vi "Insert image into excel.vi"() -> ()   [LabVIEW 2016]
panel:
  in  "error in (no error)":errorcluster
  out "error out":errorcluster
  in  "Path to image":path=path "E:/Program Files/National Instruments/LabVIEW 7.0/myStuff/test1.png"
  in  "Excel._Worksheet":refnum<k7>
  in  "Excel._Application":refnum<k7>
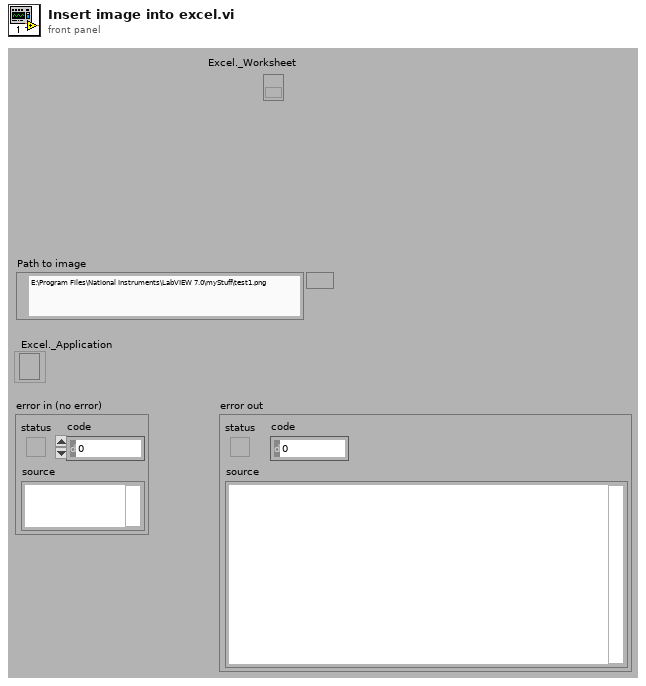
[diagram p1: front panel]
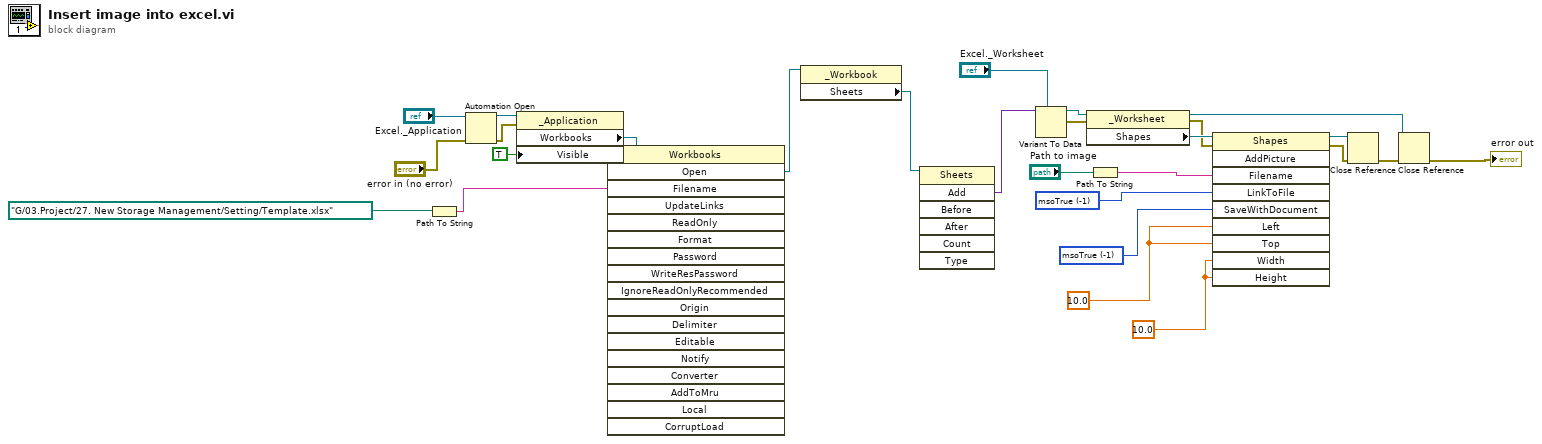
[diagram p0: block diagram]
diagram:
  w17 = -1 items=["msoTrue"=-1, "msoFalse"=0, "msoCTrue"=1, "msoTriStateToggle"=-3, "msoTriStateMixed"=-2] ("LinkToFile")
  w18 = -1 items=["msoTrue"=-1, "msoFalse"=0, "msoCTrue"=1, "msoTriStateToggle"=-3, "msoTriStateMixed"=-2] ("SaveWithDocument")
  w19 = sgl 10.0 ("Width")
  w20 = sgl 10.0 ("Left")
  n1 = Path To String(path=path "G:/03.Project/27. New Storage Management/Setting/Template.xlsx") -> (string=w1:string)
  n2 = Automation Open(error in (no error)="error in (no error)", Automation Refnum="Excel._Application") -> (Automation Refnum=w25:refnum<k7>, error out=w24:errorcluster)  [unwired: 2 in]
  n3 = property class="_Application"(reference=w25, error in=w24, "Visible"=TRUE) -> ("Workbooks"=w7:refnum<k7>)  [unwired: 2 out]
  n4 = invoke class="Workbooks" method="Open"(reference=w7, "Filename"=w1) -> ("Open"=w6:refnum<k7>)  [unwired: 16 in, 17 out]
  n5 = property class="_Workbook"(reference=w6) -> ("Sheets"=w4:refnum<k7>)  [unwired: 1 in, 2 out]
  n6 = invoke class="Sheets" method="Add"(reference=w4) -> ("Add"=w3:variant)  [unwired: 6 in, 6 out]
  n7 = Variant To Data(type="Excel._Worksheet", Variant=w3) -> (data=w10:refnum<k7>, error out=w9:errorcluster)  [unwired: 1 in]
  n8 = property class="_Worksheet"(reference=w10, error in=w9) -> (reference out=w16:refnum<k7>, error out=w14:errorcluster, "Shapes"=w22:refnum<k7>)
  n9 = Path To String(path="Path to image") -> (string=w21:string)
  n10 = invoke class="Shapes" method="AddPicture"(reference=w22, error in=w14, "Filename"=w21, "LinkToFile"=w17, "SaveWithDocument"=w18, "Left"=w20, "Top"=w20, "Width"=w19, "Height"=w19) -> (reference out=w15:refnum<k7>, error out=w13:errorcluster)  [unwired: 1 in, 8 out]
  n11 = Close Reference(reference=w15, error in (no error)=w13) -> (error out=w12:errorcluster)
  n12 = Close Reference(reference=w16, error in (no error)=w12) -> (error out=→"error out":errorcluster)
